vi "Get Subsystem Alarm Key.vi"(8 "error in (no error)":errorcluster, 10 "Active Alarm?":bool, 11 "Subsystem URL":refnum<k21>) -> (0 "error out":errorcluster, 3 "Subsystem Alarm Key":string)   [LabVIEW 2024]
doc: "Gets the key string that is used to store the control refnum in the map. The control refnum is related to alarms."
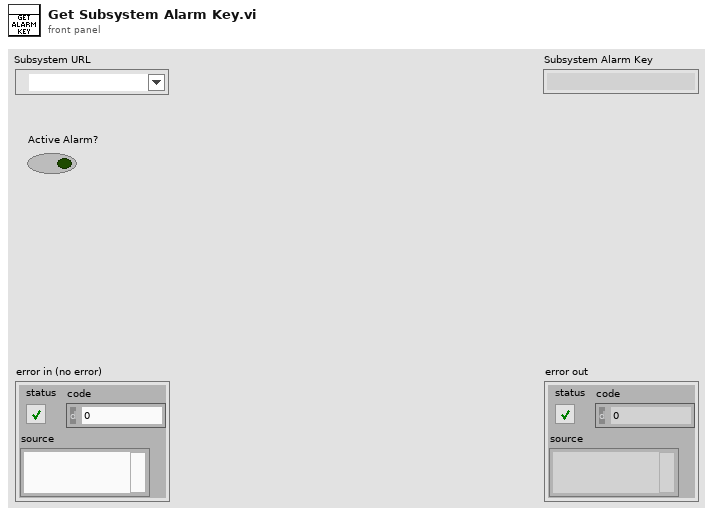
[diagram p1: front panel]
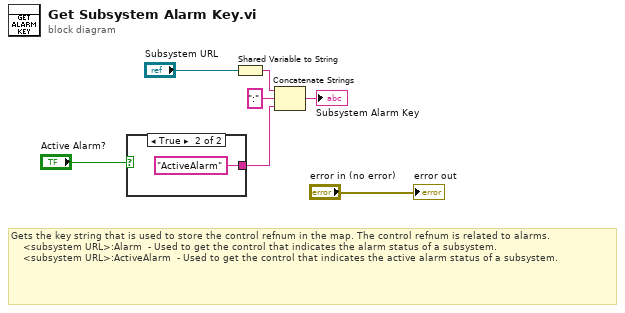
[diagram p0: block diagram]
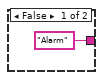
[diagram p2: hidden frame]
diagram:
  # "Gets the key string that is used to store the control refnum in the map. The control refnum is related to alarms.\n    <subsystem URL>:Alarm  - Used to get the control that indicates the alarm status of a subsystem.\n    <subsystem URL>:ActiveAlarm  - Used to get the control that indicates the active alarm status of a subsystem."
  n1 = case shown="True" "Active Alarm?" {
    tunnel: ["Alarm" ("string") "ActiveAlarm" ("string")] -> w2
    frame False {
    }
    frame True {
    }
  }
  n2 = Shared Variable to String(1:"Subsystem URL") -> (0:w1:string)
  n3 = Concatenate Strings(w1, ":" ("string"), w2) -> (→"Subsystem Alarm Key":string)
  "error out" <- "error in (no error)"
